vi "gRPC.ConvertXNETFrame.vi"(11 "frames in":T1[](array[typedef]) {"payload" format="%x"; "timestamp" format="%<%.7X\n%x>T"; "type" items=["CAN Data"=0, "CAN Remote"=1, "CAN Bus Error"=2, "CAN 2.0 Data"=8, "CAN FD Data"=16, "CAN FD+BRS Data"=24, "J1939 Data"=192, "Delay"=224, "Log Trigger"=225, "Start Trigger"=226]; "identifier" format="%x"}) -> (3 "Array":T3[](array[typedef]))   [LabVIEW 2025, in "bus_monitor_server_do.lvlib"]
uses:
  bus_monitor_server_do.lvlib
  bus_monitor_server/RPC Messages/ni_bus_monitor_api_Frame.ctl
  <vilib>/xnet/xnet.llb/XNET Frame CAN.ctl
  <vilib>/xnet/xnet.llb/XNET Frame Type CAN.ctl
  bus_monitor_server/bus_monitor_server.lvlib
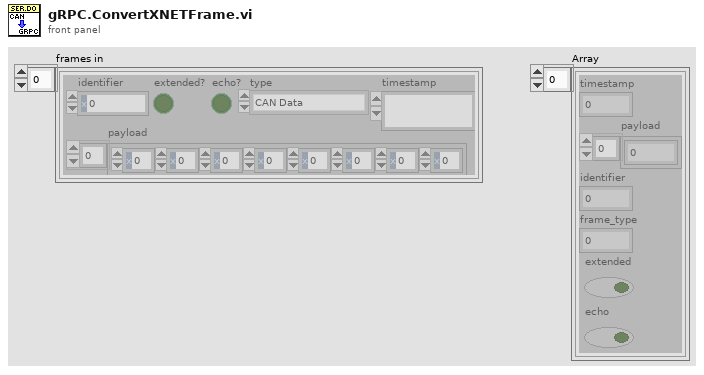
[diagram p1: front panel]
types:
  T1 = typedef "XNET Frame CAN.ctl" = cluster{"timestamp":timestamp, "payload":u8[], "identifier":u32, "type":T2, "extended?":bool, "echo?":bool}
  T2 = typedef "XNET Frame Type CAN.ctl" = u8
  T3 = typedef "bus_monitor_server.lvlib/ni_bus_monitor_api_Frame.ctl" = cluster{"timestamp":dbl, "payload":u8[], "identifier":u32, "frame_type":u32, "extended":bool, "echo":bool}
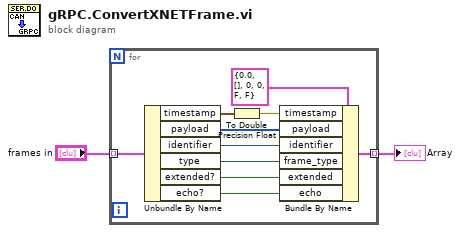
[diagram p0: block diagram]
diagram:
  n1 = for {
    tunnel: "frames in" -> [w12] mode=indexing
    tunnel: [w3] -> w2 mode=indexing
    n2 = Unbundle By Name(w12) -> ("timestamp"=w10:timestamp, "payload"=w8:u8[], "identifier"=w7:u32, "type"=w6:T2, "extended?"=w5:bool, "echo?"=w4:bool)
    n3 = To Double Precision Float(number=w10) -> (double precision float=w9:dbl)
    n4 = Bundle By Name(cluster=T3 {"timestamp"=0.0, "payload"=[], "identifier"=0, "frame_type"=0, "extended"=FALSE, "echo"=FALSE} ("ni_xnet_can_bm_api_Frame"), "timestamp"=w9, "payload"=w8, "identifier"=w7, "frame_type"=w6, "extended"=w5, "echo"=w4) -> (w3:T3)
  }
  "Array" <- w2
